vi "distance_processing.vi"(0 "Trace info in":T3, 2 "Time Stamp":timestamp, 5 "Config":T7={"IO params"={"Conversion"={"Rate"=4.0, "Num cards"=2, "Out channels"=4}, "Carriers"={"Phase shift"=180.0, "Levels"=[[0.8, 0.8, 0.8], [0.03, 0.03, 0.03]], "Delay samples"=73.15}, "TCP"={"Host"="192.168.1.15", "Port"=6666, "Buffering"=6, "Timeout"=6}, "Input channel sign"=[1, 1, 1]}, "High rate STFT"={"Win param"=101.5, "Window type"=61, "Win order"=2, "DFT size"=64, "Channels"=[7], "Oversample"=64}, "Low rate STFT"={"Win param"=120.0, "Window type"=61, "Win order"=8, "DFT size"=64, "Channels"=[7], "Oversample"=64}, "Filtering "=[]} {"Filtering"."Distortion"."Limit" format="%#_3p"; "Filtering"."Distortion"."LF cut" format="%#_3p"; "Filtering"."Kalman"."Measure noise" format="%#_3p"; "Filtering"."Kalman"."Process noise" format="%#_3p"; "Filtering"."Hum"."Limit" format="%#_3p"; "Filtering"."Hum"."Frequency" format="%#_4p"; "Low rate STFT"."Oversample" min=1 step=1; "Low rate STFT"."Channels" min=0 step=1; "Low rate STFT"."DFT size" min=1 step=1; "Low rate STFT"."Window type" items=["Rectangle"=0, "Hanning"=1, "Hamming"=2, "Blackman-Harris"=3, "Exact Blackman"=4, "Blackman"=5, "Flat Top"=6, "4 Term B-Harris "=7, "7 Term B-Harris"=8, "Low Sidelobe"=9, "Blackman Nuttall"=11, "Triangle"=30, "Bartlett-Hanning"=31, "Bohman"=32, "Parzen"=33, "Welch"=34, "Kaiser"=60, "Dolph-Chebyshev"=61, "Gaussian"=62]; "High rate STFT"."Oversample" min=1 step=1; "High rate STFT"."Channels" min=0 step=1; "High rate STFT"."DFT size" min=1 step=1; "High rate STFT"."Window type" items=["Rectangle"=0, "Hanning"=1, "Hamming"=2, "Blackman-Harris"=3, "Exact Blackman"=4, "Blackman"=5, "Flat Top"=6, "4 Term B-Harris "=7, "7 Term B-Harris"=8, "Low Sidelobe"=9, "Blackman Nuttall"=11, "Triangle"=30, "Bartlett-Hanning"=31, "Bohman"=32, "Parzen"=33, "Welch"=34, "Kaiser"=60, "Dolph-Chebyshev"=61, "Gaussian"=62]; "IO params"."Input channel sign" min=-1 max=1 step=1; "IO params"."Carriers"."Levels" min=0.0 step=0.1; "IO params"."Conversion"."Rate" format="%#_8g"}, 6 "Carrier amplitudes":T6 format="%#_3p", 10 "Output options":T1={"Source"=enum."X", "Sensor"=enum."X", "Sense"=FALSE, "Distance"=FALSE, "LF corner"=0.1, "RMS Tc"=5.0}, 11 "Modulation info":T15={"Fs full"=0.0, "Fs high"=0.0, "Fs low"=0.0, "Read size"=0, "FFT size low"=5000, "df low"=5000.0, "High carriers"=[], "Low carriers"=[], "Hi channels at low"=[7]} {"Hi channels at low" min=0 step=1; "Low carriers" format="%#_6p"; "High carriers" format="%#_6p"}, 12 "Calibration":T13 {"r bias" format="%_3p"; "Ks" format="%#_3p"}, 13 "Reset":bool, 15 "Reset RMS":bool, 16 "Measurements In":T16 {"RMS" format="%#_3p"; "Relative" format="%.4f"; "Ref distance" format="%.3f"; "DC" format="%.3f"}, 17 "High carrier amplitudes":T14 format="%#_3p") -> (20 "Measurements out":T16 {"RMS" format="%#_3p"; "Relative" format="%.4f"; "Ref distance" format="%.3f"; "DC" format="%.3f"}, 22 "Mean level":dbl[](array[numeric]), 23 "Chart display":waveform(dbl)[](array[waveform]), 26 "Trace info out":T3)   [LabVIEW 2026]
uses:
  gui/measurements.ctl
  processing/modulation_info.ctl
  processing/high_carrier_amplitudes.ctl
  calibration.ctl
  processing/ilemt_config.ctl
  system/IO_params.ctl
  processing/stft_params.ctl
  <vilib>/Analysis/4window.llb/windowTd.ctl
  processing/filter_params.ctl
  processing/detrend_mode.ctl
  processing/carrier_amplitudes.ctl
  gui/trace_info.ctl
  gui/trace_channel.ctl
  main/ilemt_status.ctl
  gui/output_options.ctl
  gui/coupling_selector.ctl
  main/ilemt_globals.vi
  <vilib>/Analysis/NI_AALPro.lvlib
panel:
  # "This is an input (as well as an output) because this is where we keep the reference distance."
  # "This is used by the builtin 1DOF calibration"
  # "High rate time samples of high carrier amplitudes"
  # "Low rate measurement of all carrier amplitudes"
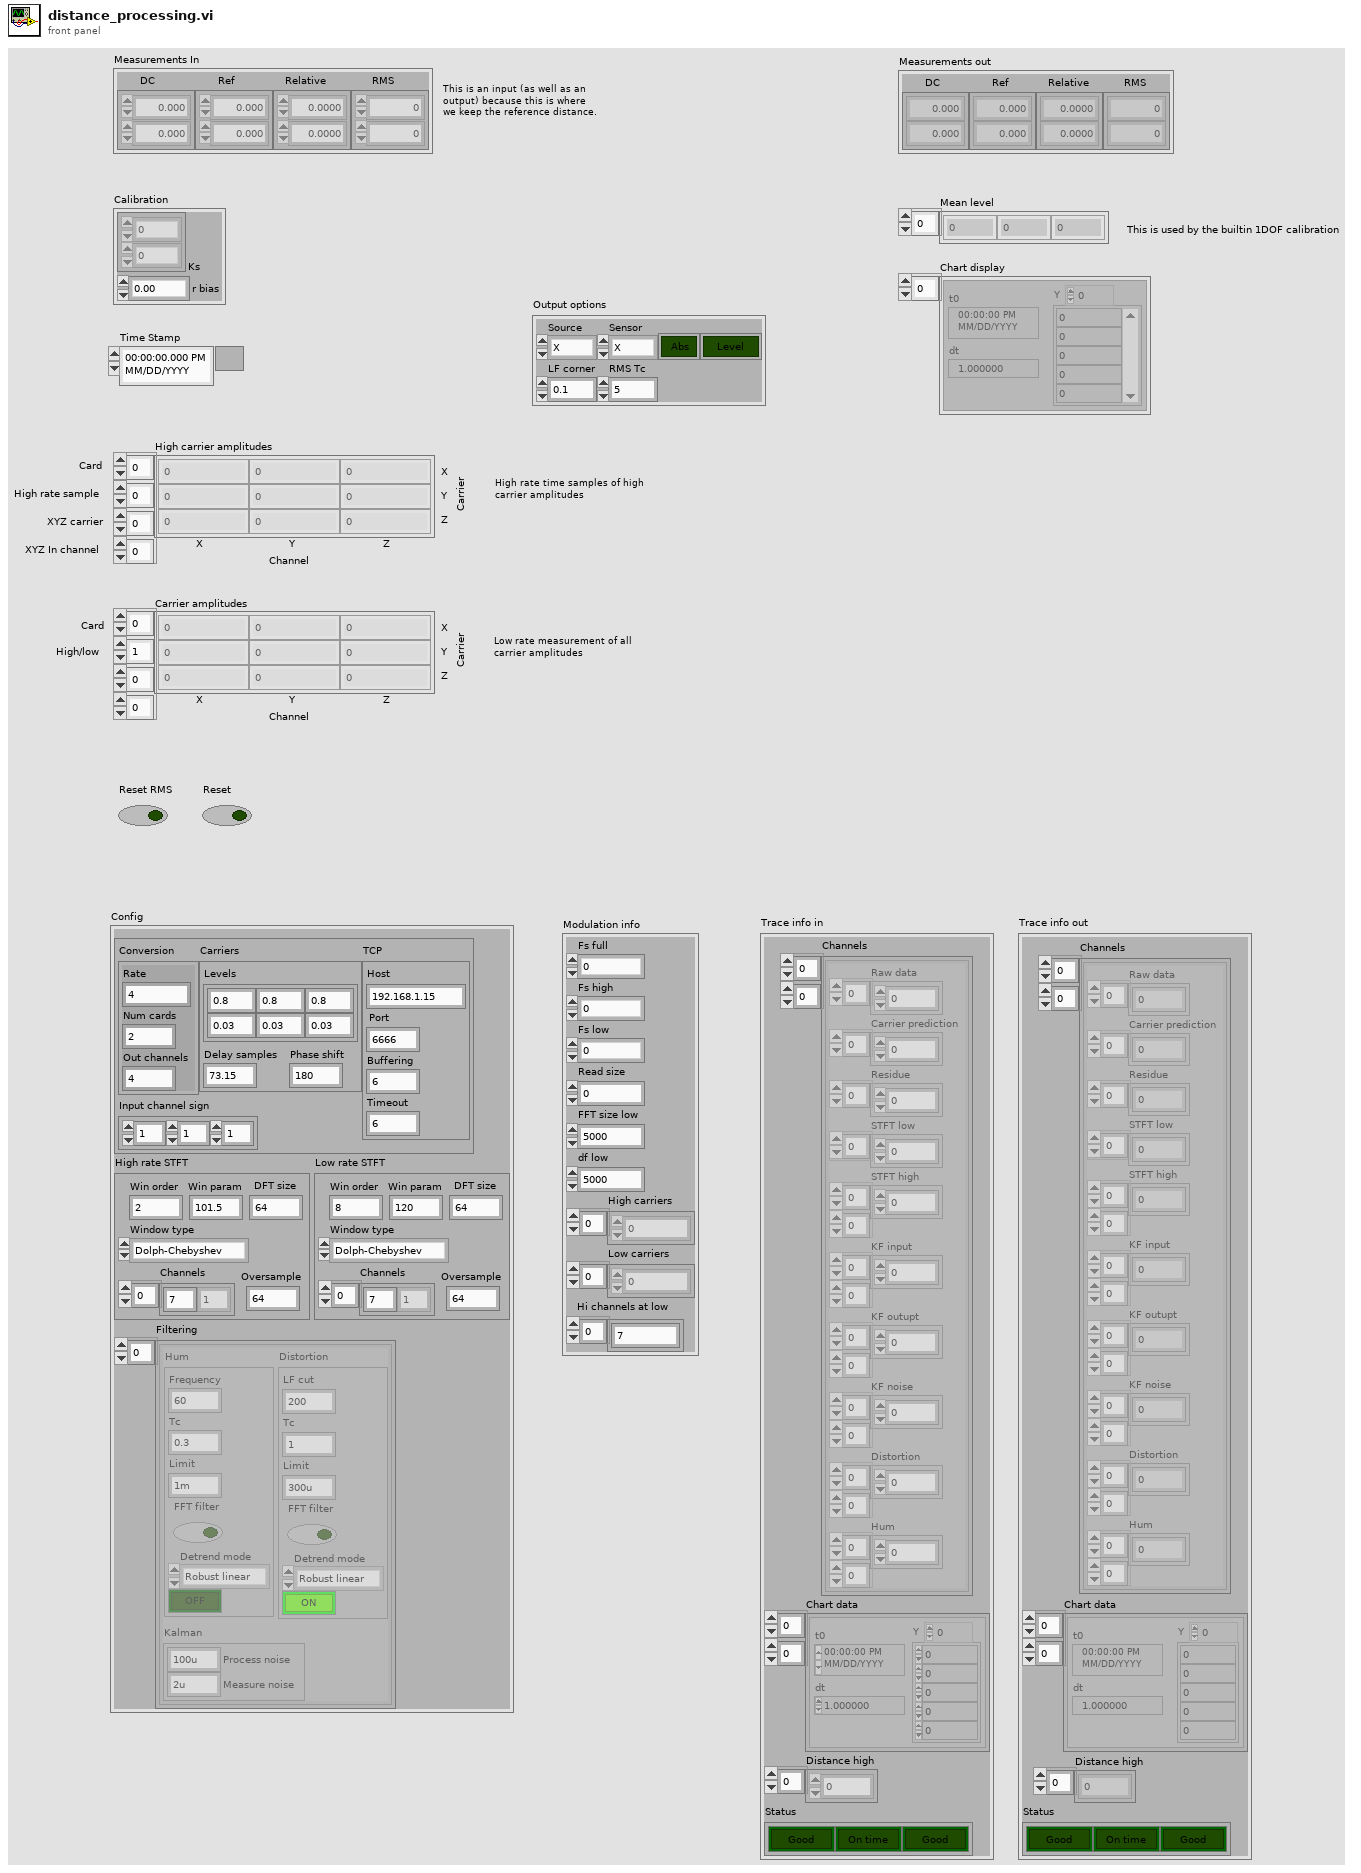
[diagram p1: front panel]
types:
  T1 = typedef "output_options.ctl" = cluster{"Source":T2, "Sensor":T2, "Sense":bool, "Distance":bool, "LF corner":dbl, "RMS Tc":dbl}
  T2 = typedef "coupling_selector.ctl" = enum16{"X", "Y", "Z", "Vector"}
  T3 = typedef "trace_info.ctl" = cluster{"Channels":T4[][], "Chart data":waveform(dbl)[][], "Distance high":dbl[], "Status":T5}
  T4 = typedef "trace_channel.ctl" = cluster{"Raw data":dbl[], "Carrier prediction":dbl[], "Residue":dbl[], "STFT low":cdb[], "STFT high":cdb[][], "KF input":cdb[][], "KF outupt":cdb[][], "KF noise":dbl[][], "Distortion":cdb[][], "Hum":cdb[][]}
  T5 = typedef "ilemt_status.ctl" = cluster{"NaN":bool, "Backlog":bool, "Clipping":bool}
  T6 = typedef "carrier_amplitudes.ctl" = cdb[][][][]
  T7 = typedef "ilemt_config.ctl" = cluster{"IO params":T8, "High rate STFT":T9, "Low rate STFT":T9, "Filtering ":T11[]}
  T8 = typedef "IO_params.ctl" = cluster{"Conversion":cluster{"Rate":dbl, "Num cards":u32, "Out channels":u32}, "Carriers":cluster{"Phase shift":dbl, "Levels":dbl[][], "Delay samples":dbl}, "TCP":cluster{"Host":string, "Port":i32, "Buffering":u32, "Timeout":u32}, "Input channel sign":i32[]}
  T9 = typedef "stft_params.ctl" = cluster{"Win param":dbl, "Window type":T10, "Win order":i32, "DFT size":i32, "Channels":i32[], "Oversample":i32}
  T10 = typedef "NI_AALPro.lvlib/windowTd.ctl" = u32
  T11 = typedef "filter_params.ctl" = cluster{"Hum":cluster{"Frequency":dbl, "Tc":dbl, "Limit":dbl, "FFT filter":bool, "Detrend mode":T12, "Enable":bool}, "Kalman":cluster{"Process noise":dbl, "Measure noise":dbl}, "Distortion":cluster{"LF cut":dbl, "Tc":dbl, "Limit":dbl, "FFT filter":bool, "Detrend mode":T12, "Enable":bool}}
  T12 = typedef "detrend_mode.ctl" = enum16{"Zero mean", "Linear", "Robust linear"}
  T13 = typedef "calibration.ctl" = cluster{"Ks":dbl[], "r bias":dbl}
  T14 = typedef "high_carrier_amplitudes.ctl" = cdb[][][][]
  T15 = typedef "modulation_info.ctl" = cluster{"Fs full":dbl, "Fs high":dbl, "Fs low":dbl, "Read size":i32, "FFT size low":i32, "df low":dbl, "High carriers":dbl[], "Low carriers":dbl[], "Hi channels at low":i32[]}
  T16 = typedef "measurements.ctl" = cluster{"DC":dbl[], "Ref distance":dbl[], "Relative":dbl[], "RMS":dbl[]}
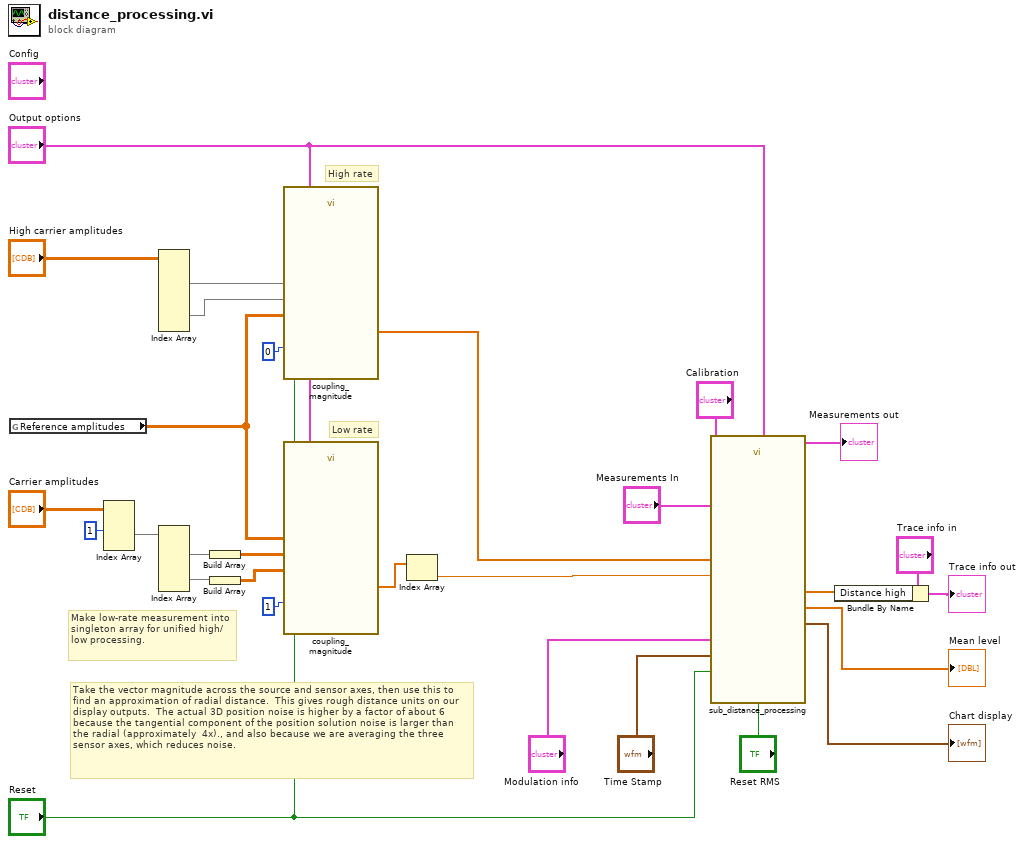
[diagram p0: block diagram]
diagram:
  # "Low rate"
  # "High rate"
  # "Make low-rate measurement into singleton array for unified high/low processing."
  # "Take the vector magnitude across the source and sensor axes, then use this to find an approximation of radial distance.  This gives rough distance units on our display outputs.  The actual 3D position noise is higher by a factor of about 6 because the tangential component of the position solution noise is larger than the radial (approximately  4x)., and also because we are averaging the three sensor axes, which reduces noise."
  n1 = global read "ilemt_globals.vi" "Reference amplitudes"() -> (w1:T6)
  n2 = Index Array(array="Carrier amplitudes", index (dim 1)=1 ("disabled index (row)")) -> (element=w8:cdb[][][])  [unwired: 3 in]
  n3 = Index Array(array="High carrier amplitudes") -> (element #1=w3:cdb[][][], element #2=w10:cdb[][][])  [unwired: 8 in]
  n4 = Index Array(array=w8) -> (element #1=w6:cdb[][], element #2=w7:cdb[][])  [unwired: 6 in]
  n5 = Build Array(w6) -> (w5:cdb[][][])
  n6 = Build Array(w7) -> (w11:cdb[][][])
  n7 = call "coupling_magnitude.vi"("Reset"="Reset", "High/low index"=0, "Ref carrier amplitudes"=w1, "Sense amplitudes"=w3, "Carrier amplitudes"=w10, "Output options"="Output options") -> ("Magnitudes"=w19:dbl[])  [unwired: 5 in]
  n8 = call "coupling_magnitude.vi"("Reset"="Reset", "High/low index"=1, "Ref carrier amplitudes"=w1, "Sense amplitudes"=w5, "Carrier amplitudes"=w11, "Output options"="Output options") -> ("Magnitudes"=w13:dbl[])  [unwired: 5 in]
  n9 = Index Array(array=w13) -> (element=w12:dbl)  [unwired: 1 in]
  n10 = call "sub_distance_processing.vi"("Magnitude high"=w19, "Calibration"="Calibration", "Measurements In"="Measurements In", "Magnitude low"=w12, "Modulation info"="Modulation info", "Reset"="Reset", "Output options"="Output options", "Reset RMS"="Reset RMS", "Time Stamp"="Time Stamp") -> ("Measurements out"=→"Measurements out":T16, "Mean level"=→"Mean level":dbl[], "Chart display"=→"Chart display":waveform(dbl)[], "Distance high"=w23:dbl[])  [unwired: 3 in]
  n11 = Bundle By Name(cluster="Trace info in", "Distance high"=w23) -> (→"Trace info out":T3)
